vi "CRYASIO Get Device Informaion.vi"(11 "error in (no error)":errorcluster) -> (4 "ASIO Output Device Infor":T1(array[cluster]), 6 "ASIO Output Device Name":string[](array[string]), 8 "ASIO Input Device Infor":T1(array[cluster]), 10 "ASIO Input Device Name":string[](array[string]), 15 "error out":errorcluster)   [LabVIEW 2013]
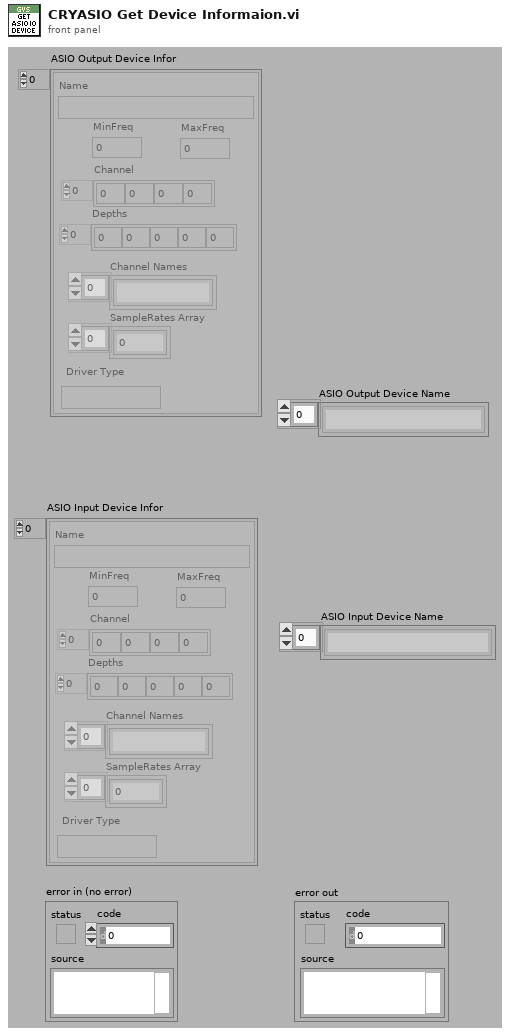
[diagram p1: front panel]
types:
  T1 = cluster{"Name":string, "MinFreq":dbl, "MaxFreq":dbl, "Channel":i32[], "Depths":i32[], "Channel Names":string[], "SampleRates Array":dbl[], "Driver Type":string}[]
  T2 = cluster{"Name":string, "MinFreq":dbl, "MaxFreq":dbl, "Channel":i32[], "Depths":i32[], "Channel Names":string[], "SampleRates Array":dbl[], "Driver Type":string}
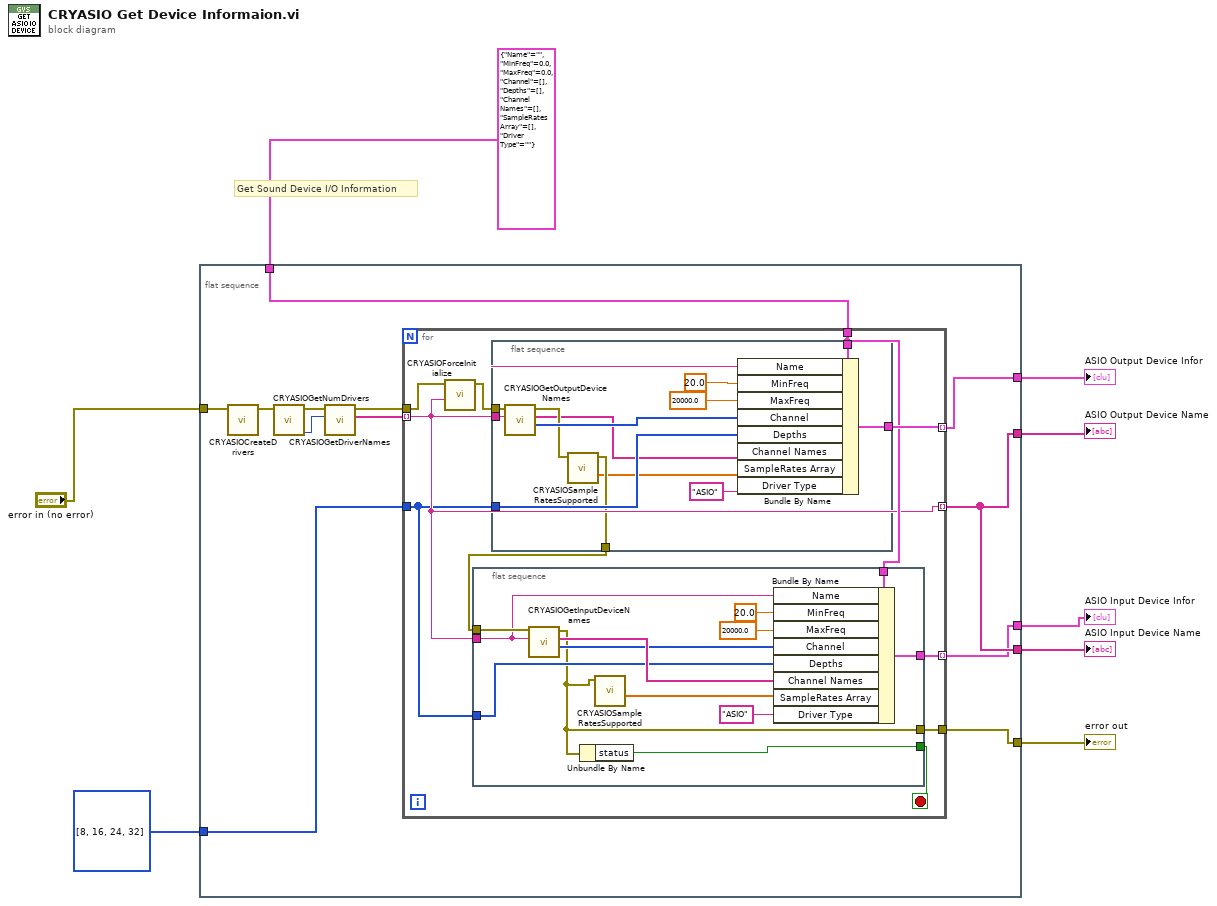
[diagram p0: block diagram]
diagram:
  # "Get Sound Device I/O Information"
  n1 = flat-sequence {
    tunnel: [w11] -> w7
    tunnel: [w9] -> w8
    tunnel: [w14] -> w6
    tunnel: [w10] -> w5
    tunnel: [w11] -> w4
    tunnel: T2 {"Name"="", "MinFreq"=0.0, "MaxFreq"=0.0, "Channel"=[], "Depths"=[], "Channel Names"=[], "SampleRates Array"=[], "Driver Type"=""} ("I_Device Infor") -> [w15]
    tunnel: i32[] [8, 16, 24, 32] ("Depths") -> [w13]
    tunnel: "error in (no error)" -> [w12]
    frame #0 {
      n2 = call "CRYASIOCreateDrivers.vi"("error in (no error)"=w12) -> ("error out"=w19:errorcluster)  [unwired: 10 in]
      n3 = call "CRYASIOGetNumDrivers.vi"("error in (no error)"=w19) -> ("Drive Num"=w20:i32, "error out"=w18:errorcluster)  [unwired: 9 in]
      n4 = call "CRYASIOGetDriverNames.vi"("Driver Count"=w20, "error in (no error)"=w18) -> ("Driver Name Array"=w17:string[], "error out"=w16:errorcluster)  [unwired: 8 in]
      n5 = for {
        tunnel: w13 -> [w21]
        tunnel: w17 -> [w25] mode=indexing
        tunnel: w16 -> [w28]
        tunnel: w15 -> [w27]
        tunnel: [w30] -> w14 mode=indexing
        tunnel: [w25] -> w11 mode=indexing
        tunnel: [w26] -> w10 mode=indexing
        tunnel: [w22] -> w9
        stop <- w23 stop-if-true
        n6 = call "CRYASIOForceInitialize.vi"("Driver Name"=w25, "error in (no error)"=w28) -> ("error out"=w29:errorcluster)  [unwired: 8 in, 1 out]
        n7 = flat-sequence {
          tunnel: [w43] -> w23
          tunnel: w21 -> [w40]
          tunnel: w27 -> [w37]
          tunnel: w24 -> [w35]
          tunnel: [w34] -> w26
          tunnel: [w33] -> w22
          tunnel: w25 -> [w31]
          frame #0 {
            n8 = call "CRYASIOGetInputDeviceNames.vi"("Driver Name"=w31, "error in (no error)"=w35) -> ("Channel Idx"=w41:u32[], "Output Device Names"=w42:string[], "error out"=w33:errorcluster)  [unwired: 7 in]
            n9 = Unbundle By Name(w33) -> ("status"=w43:bool)
            n10 = call "CRYASIOSampleRatesSupported.vi"("error in (no error)"=w33) -> ("SampleRates Array"=w32:dbl[])  [unwired: 8 in, 2 out]
            n11 = Bundle By Name(cluster=w37, "Name"=w31, "MinFreq"=20.0, "MaxFreq"=20000.0, "Channel"=w41, "Depths"=w40, "Channel Names"=w42, "SampleRates Array"=w32, "Driver Type"="ASIO") -> (w34:T2)
          }
        }
        n12 = flat-sequence {
          tunnel: w21 -> [w56]
          tunnel: w27 -> [w52]
          tunnel: [w49] -> w24
          tunnel: [w48] -> w30
          tunnel: w29 -> [w45]
          tunnel: w25 -> [w44]
          frame #0 {
            n13 = call "CRYASIOGetOutputDeviceNames.vi"("Driver Name"=w44, "error in (no error)"=w45) -> ("Channel Idx"=w55:u32[], "Output Device Names"=w47:string[], "error out"=w50:errorcluster)  [unwired: 7 in]
            n14 = call "CRYASIOSampleRatesSupported.vi"("error in (no error)"=w50) -> ("SampleRates Array"=w46:dbl[], "error out"=w49:errorcluster)  [unwired: 8 in, 1 out]
            n15 = Bundle By Name(cluster=w52, "Name"=w44, "MinFreq"=20.0, "MaxFreq"=20000.0, "Channel"=w55, "Depths"=w56, "Channel Names"=w47, "SampleRates Array"=w46, "Driver Type"="ASIO") -> (w48:T2)
          }
        }
      }
    }
  }
  "ASIO Output Device Infor" <- w6
  "ASIO Input Device Infor" <- w5
  "error out" <- w8
  "ASIO Output Device Name" <- w7
  "ASIO Input Device Name" <- w4
